vi "44.vi"() -> ()   [LabVIEW 2021]
uses:
  4a520fb6-f452-43af-9724-12665c221796.vi
  <vilib>/Comparison/Less/Less Functor/Less Functor.lvclass
panel:
  out "Array":u64[](array[numeric])
  in  "Numeric":i32=10000
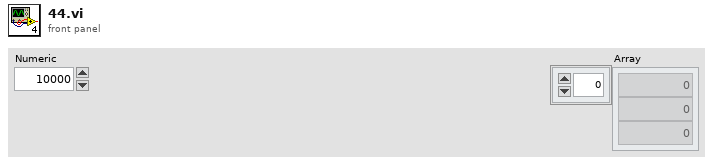
[diagram p1: front panel]
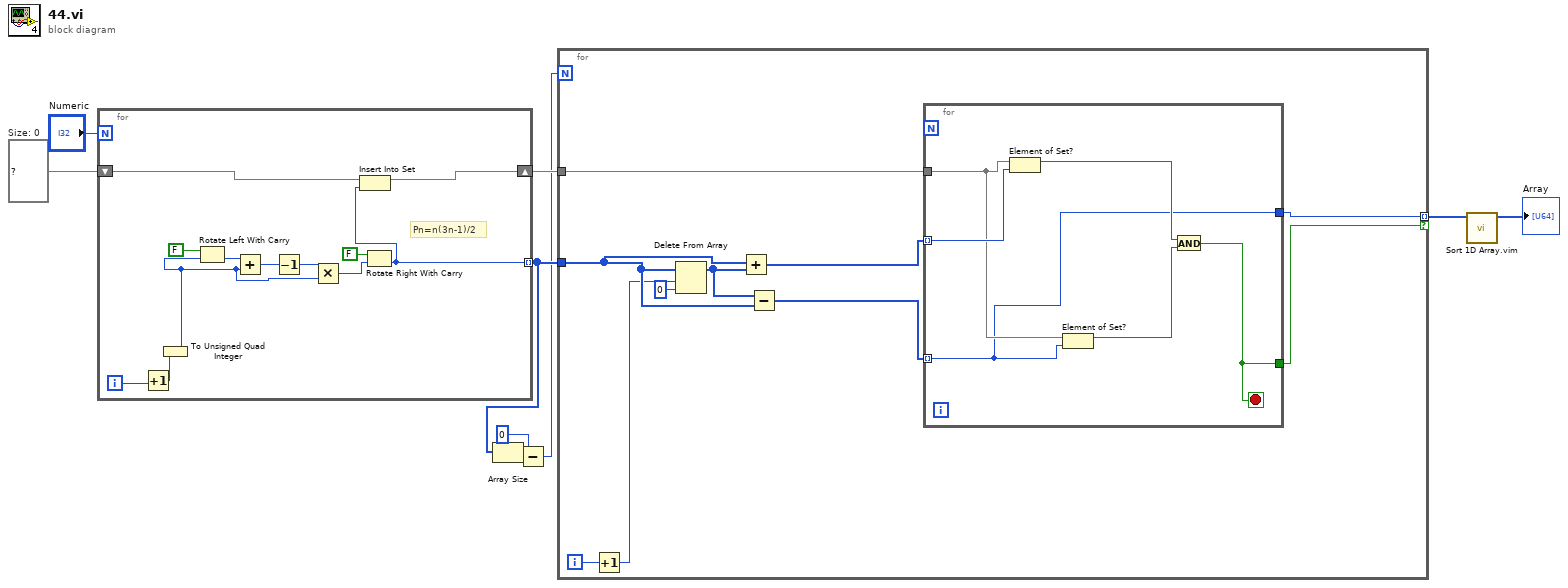
[diagram p0: block diagram]
diagram:
  w8 = set{u64} {}  # Size: 0
  n1 = for {
    N: "Numeric" -> [_]
    shift-right: [w13] -> w7
    shift-left: w8 -> [w12]
    tunnel: [w11] -> w6 mode=indexing
    i -> [w21]
    # "Pn=n(3n-1)/2"
    n2 = Increment(x=w21) -> (x+1=w14:i32)
    n3 = To Unsigned Quad Integer(1:w14) -> (0:w10:u64)
    n4 = Rotate Left With Carry(2:w10, 3:FALSE ("carry")) -> (0:w15:u64)  [unwired: 1 out]
    n5 = Add(x=w15, y=w10) -> (x+y=w19:u64)
    n6 = Decrement(x=w19) -> (x-1=w18:u64)
    n7 = Multiply(x=w18, y=w10) -> (x*y=w16:u64)
    n8 = Rotate Right With Carry(2:w16, 3:FALSE ("carry")) -> (0:w11:u64)  [unwired: 1 out]
    n9 = Insert Into Set(10:w11, 11:w12) -> (3:w13:set{u64})  [unwired: 1 out]
  }
  n10 = Array Size(array=w6) -> (size(s)=w5:i32)
  n11 = Subtract(x=w5, y=0) -> (x-y=w4:i32)
  n12 = for {
    N: w4 -> [_]
    tunnel: w6 -> [w30]
    tunnel: w7 -> [w26]
    tunnel: [w23] -> w2 mode=indexing if=w22
    i -> [w25]
    n13 = Increment(x=w25) -> (x+1=w24:i32)
    n14 = Delete From Array(array=w30, length=w24, index=0) -> (array with subset deleted=w31:u64[])  [unwired: 1 out]
    n15 = Add(x=w30, y=w31) -> (x+y=w27:u64[])
    n16 = Subtract(x=w31, y=w30) -> (x-y=w28:u64[])
    n17 = for {
      tunnel: w28 -> [w32] mode=indexing
      tunnel: w27 -> [w37] mode=indexing
      tunnel: w26 -> [w36]
      tunnel: [w33] -> w22
      tunnel: [w32] -> w23
      stop <- w33 stop-if-true
      n18 = Element of Set?(10:w37, 11:w36) -> (3:w35:bool)
      n19 = Element of Set?(10:w32, 11:w36) -> (3:w34:bool)
      n20 = And(x=w35, y=w34) -> (x .and. y?=w33:bool)
    }
  }
  n21 = call "Sort 1D Array.vim"("unsorted array"=w2) -> ("sorted array"=→"Array":u64[])  [unwired: 10 in]
